vi "cpu.vi"() -> ()   [LabVIEW 2019]
uses:
  <resource>/objmgr/ni.dex.rc
panel:
  out "error out 5":errorcluster
  out "error out 4":errorcluster
  in  "stop":bool
  out "Connected":bool
  out "Waveform Chart":dbl(graph)
  out "error out 2":errorcluster
  out "error out":errorcluster
  out "error out 3":errorcluster
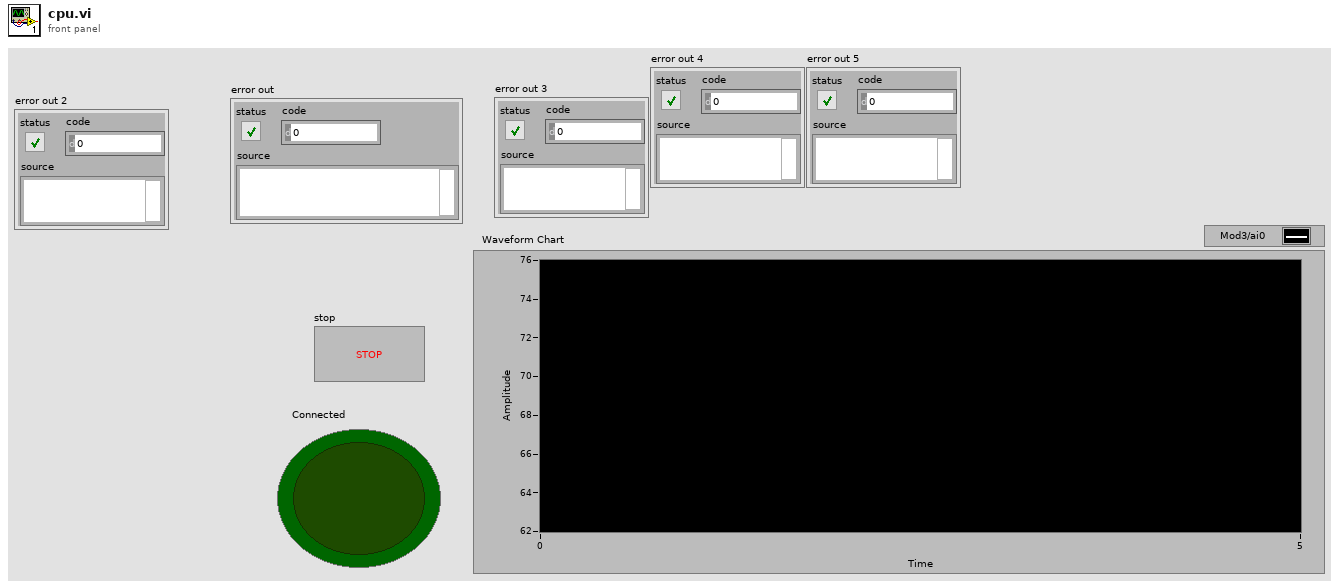
[diagram p1: front panel]
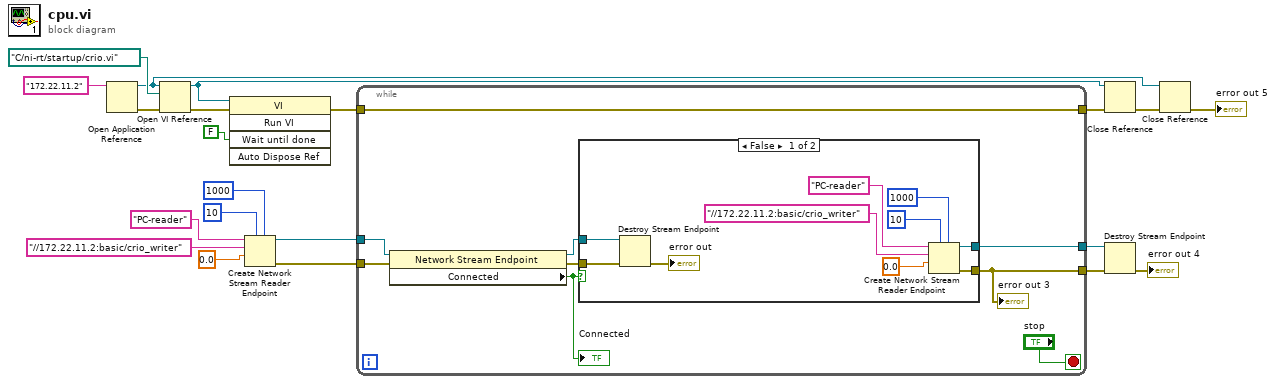
[diagram p0: block diagram]
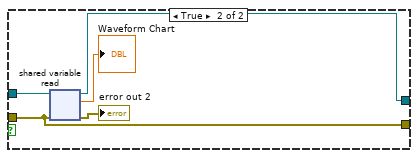
[diagram p2: hidden frame]
diagram:
  n1 = Open Application Reference(11:"172.22.11.2" ("machine name (\"\":  open local reference)")) -> (0:w9:errorcluster, 3:w2:refnum<vi>)  [unwired: 3 in]
  n2 = Open VI Reference(application reference (local)=w2, vi path=path "C:/ni-rt/startup/crio.vi", error in (no error)=w9) -> (vi reference=w4:refnum<vi>, error out=w8:errorcluster)  [unwired: 3 in]
  n3 = invoke class="VI" method="Run VI"(reference=w4, error in=w8, "Wait until done"=FALSE ("Wait Until Done")) -> (error out=w5:errorcluster)  [unwired: 2 in, 4 out]
  n4 = Create Network Stream Reader Endpoint(5:1000 ("timeout in ms (-1)"), 7:10 ("reader buffer size"), 9:0.0, 10:"//172.22.11.2:basic/crio_writer" ("writer url"), 11:"PC-reader" ("reader name")) -> (0:w15:errorcluster, 3:w16:refnum<k21>)  [unwired: 2 in]
  n5 = while {
    tunnel: w15 -> [w25]
    tunnel: [w23] -> w13
    tunnel: w16 -> [w29]
    tunnel: [w24] -> w14
    tunnel: [w22] -> w6
    tunnel: w5 -> [w22]
    stop <- "stop" stop-if-true
    n6 = property class="Network Stream Endpoint"(reference=w29, error in=w25) -> (reference out=w28:refnum<k21>, error out=w26:errorcluster, "Connected"=w27:bool)
    "Connected" <- w27
    n7 = case shown="False" w27 {
      tunnel: w28 -> [w40 w42]
      tunnel: w26 -> [w39 w43]
      tunnel: [w33 w45] -> w24
      tunnel: [w32 w43] -> w23
      frame False {
        n8 = Destroy Stream Endpoint(8:w39, 11:w40) -> (0:→"error out":errorcluster)
        n9 = Create Network Stream Reader Endpoint(5:1000 ("timeout in ms (-1)"), 7:10 ("reader buffer size"), 9:0.0, 10:"//172.22.11.2:basic/crio_writer" ("writer url"), 11:"PC-reader" ("reader name")) -> (0:w32:errorcluster, 3:w33:refnum<k21>)  [unwired: 2 in]
      }
      frame True {
        n10 = shared-variable-read(w42, w43) -> (w45:refnum<k21>, →"error out 2":errorcluster, →"Waveform Chart":dbl)  [unwired: 1 in, 1 out]
      }
    }
    "error out 3" <- w23
  }
  n11 = Close Reference(reference=w4, error in (no error)=w6) -> (error out=w3:errorcluster)
  n12 = Destroy Stream Endpoint(8:w13, 11:w14) -> (0:→"error out 4":errorcluster)
  n13 = Close Reference(reference=w2, error in (no error)=w3) -> (error out=→"error out 5":errorcluster)
